vi "Read Parameters to process.vi"(8 "error in":errorcluster, 11 "BuckBoost runtime in":refnum<class "BuckBoost runtime.lvclass">) -> (0 "error out":errorcluster, 2 "Parameters to process":T1, 3 "BuckBoost runtime out":refnum<class "BuckBoost runtime.lvclass">)   [LabVIEW 2017, in "BuckBoost runtime.lvclass"]
uses:
  BuckBoost runtime.lvclass
  configuration/parameter data indices.ctl
  BuckBoost runtime.lvclass/BuckBoost runtime.ctl
  configuration/BuckBoost configuration.lvclass
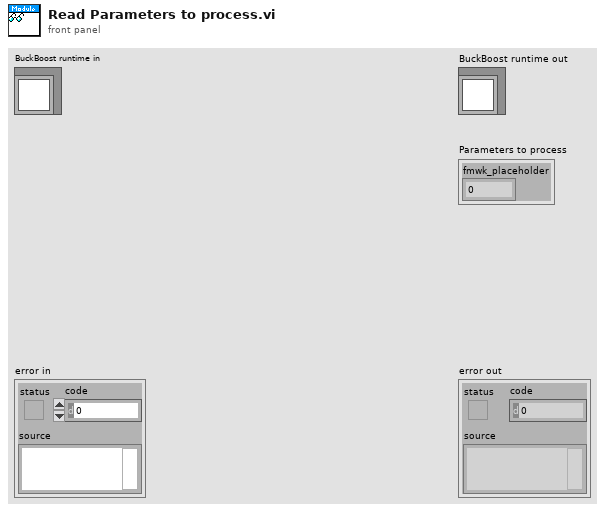
[diagram p1: front panel]
types:
  T1 = typedef "BuckBoost configuration.lvclass/parameter data indices.ctl" = cluster{"fmwk_placeholder":i32}
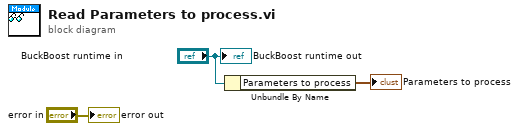
[diagram p0: block diagram]
diagram:
  n1 = Unbundle By Name("BuckBoost runtime in") -> ("Parameters to process"=→"Parameters to process":T1)
  "error out" <- "error in"
  "BuckBoost runtime out" <- "BuckBoost runtime in"
